vi "Datasocket(多个信号)客户机.vi"() -> ()   [LabVIEW 2017]
panel:
  in  "停止":bool
  out "波形图":dbl[](graph)
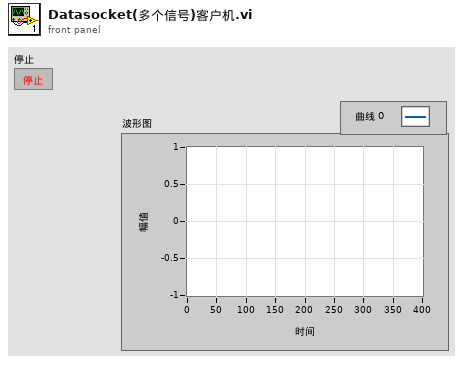
[diagram p1: front panel]
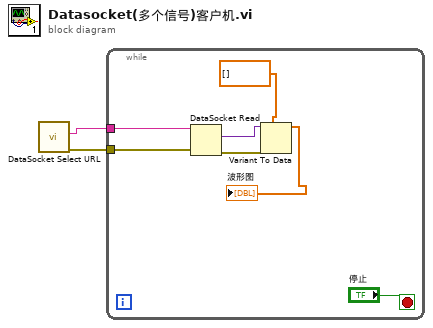
[diagram p0: block diagram]
diagram:
  n1 = call <vilib>:"DataSocket Select URL.vi"() -> ("error out"=w1:errorcluster, "URL"=w2:string)  [unwired: 9 in, 1 out]
  n2 = while {
    tunnel: w2 -> [w9]
    tunnel: w1 -> [w8]
    stop <- "停止" stop-if-true
    n3 = DataSocket Read(8:w8, 11:w9) -> (0:w7:errorcluster, 2:w3:variant)  [unwired: 3 in, 5 out]
    n4 = Variant To Data(error in=w7, type=dbl[] [], Variant=w3) -> (data=→"波形图":dbl[])  [unwired: 1 out]
  }
